vi "run_experiment_sCMOS_DAC_DEBUG_WORKING_INTER.vi"() -> ()   [LabVIEW 2015]
uses:
  <vilib>/DAQmx/read.llb/DAQmx Read (Analog 1D Wfm NChan NSamp).vi
  <vilib>/DAQmx/write.llb/DAQmx Write (Digital Bool 1Line 1Point).vi
  <vilib>/DAQmx/create/channels.llb/DAQmx Create Channel (DO-Digital Output).vi
  <vilib>/DAQmx/miscellaneous.llb/DAQmx Fill In Error Info.vi
  <vilib>/DAQmx/create/channels.llb/DAQmx Create Channel (AI-Voltage-Basic).vi
  <vilib>/DAQmx/configure/timing.llb/DAQmx Timing (Sample Clock).vi
panel:
  out "Display":T1(plugin-control)
  out "DAC Input":waveform(dbl)[](graph) caption="DAC Input Display"
  out "error out":errorcluster
  out "Current Stimulus Name":string
  out "Current Piezo Command":dynamicdata(graph)
  out "Acquiring Frames":bool
  out "Current Stim Duration":dbl
  out "Current Stimulus Save Path":path
  in  "Number Reps":dbl
  out "Experiment Path":path
  out "Timestamp":string
  out "Genotype":string
  out "Fly Name":string
  out "Experiment Name":string
  in  "Metadata Path":path
  out "Stimulus Files":path[](array[path])
  out "Num Stimuli":i32
  out "Protocol Name":string
  out "Protocol Rate":i32
  in  "Protocol Path":path
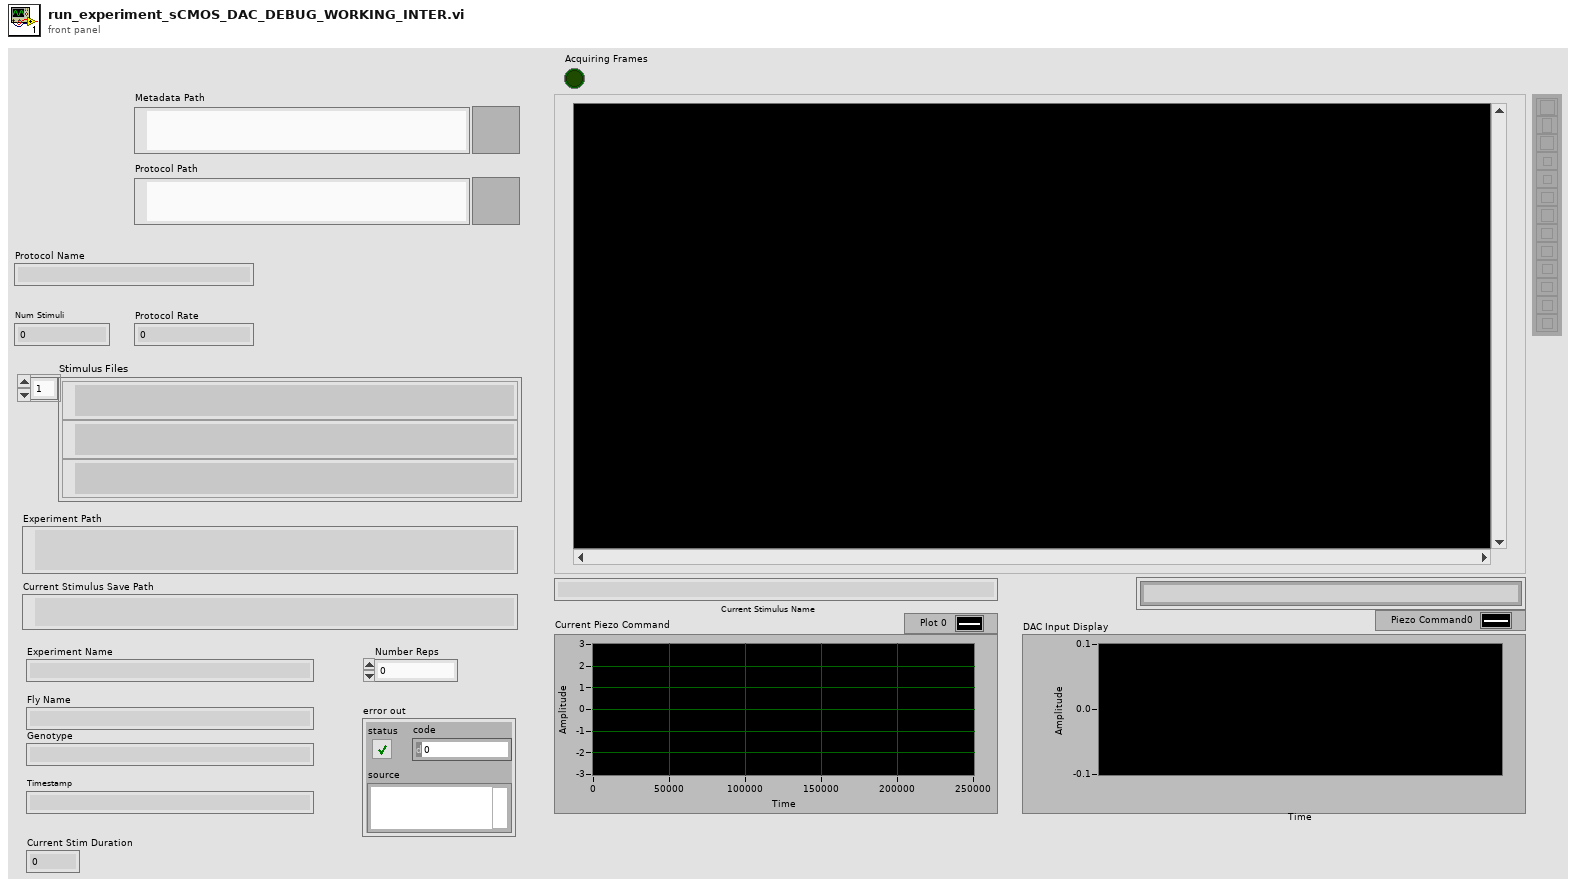
[diagram p1: front panel]
types:
  T1 = typedef "IMAQ Image.ctl" = refnum<image>
  T2 = cluster{"Value":i32, "Minimum":i32, "Maximum":i32, "Increment":i32}
  T3 = cluster{"height":u32, "width":u32, "datatype":u32}
  T4 = typedef "Image Type" = u32
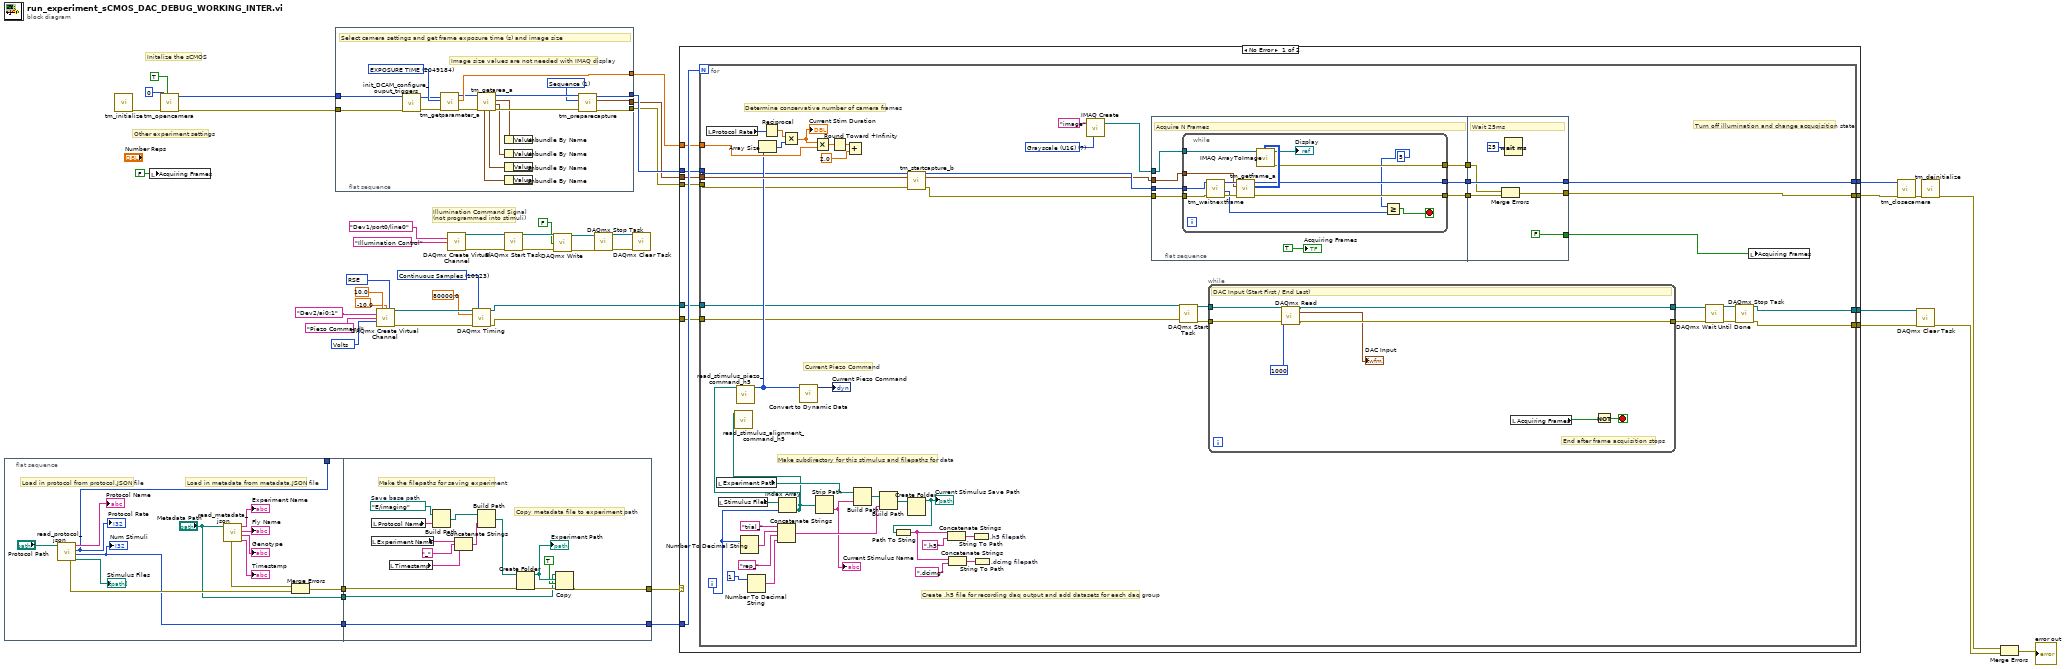
[diagram p0: block diagram]
diagram:
  w8 = 10083 items=["default"=-1, "RSE"=10083, "NRSE"=10078, "Differential"=10106, "Pseudodifferential"=12529] ("input terminal configuration")
  w9 = 10123 items=["Finite Samples"=10178, "Continuous Samples"=10123] ("sample mode")
  w10 = 10348 items=["Volts"=10348, "From Custom Scale"=10065] ("units")
  # "Other experiment settings"
  # "Initalize the sCMOS"
  # "Illumination Command Signal \n(not programmed into stimuli)"
  n1 = flat-sequence {
    tunnel: [w49] -> _
    tunnel: [w50] -> w21
    tunnel: ["Metadata Path"] -> w20
    tunnel: [w47] -> w19
    tunnel: [w74] -> w40
    tunnel: w21 -> [w62]
    tunnel: w20 -> [w61]
    tunnel: w19 -> [w74]
    tunnel: [w60] -> w18
    frame #0 {
      # "Load in metadata from metadata.JSON file"
      # "Load in protocol from protocol.JSON file"
      n2 = call "read_protocol_json.vi"("Path"="Protocol Path") -> ("stims"=→"Stimulus Files":path[], "n_stims"=w47:i32, "rate"=w49:i32, "protocol name"=→"Protocol Name":string, "error out"=w52:errorcluster)  [unwired: 6 in]
      "Protocol Rate" <- w49
      "Num Stimuli" <- w47
      n3 = call "read_metadata_json.vi"("Path"="Metadata Path") -> ("exp_time"=→"Timestamp":string, "genotype"=→"Genotype":string, "fly_name"=→"Fly Name":string, "exp_ name"=→"Experiment Name":string, "error out"=w51:errorcluster)  [unwired: 6 in]
      n4 = Merge Errors(w51, w52) -> (w50:errorcluster)
    }
    frame #1 {
      w69 = path "E:/imaging"  # Save base path
      # "Copy metadata file to experiment path"
      # "Make the filepaths for saving experiment"
      n5 = local read "Experiment Name"() -> (w66:string)
      n6 = local read "Protocol Name"() -> (w68:string)
      n7 = local read "Timestamp"() -> (w64:string)
      n8 = Build Path(base path=w69, name or relative path=w68) -> (appended path=w67:path)
      n9 = Concatenate Strings(w66, "_", w64) -> (w63:string)
      n10 = Build Path(base path=w67, name or relative path=w63) -> (appended path=w70:path)
      n11 = Create Folder(path (use dialog)=w70, error in=w62) -> (created path=w73:path, error out=w72:errorcluster)  [unwired: 1 in, 1 out]
      "Experiment Path" <- w73
      n12 = Copy(8:w72, 9:TRUE ("overwrite (F)"), 10:w73, 11:w61) -> (0:w60:errorcluster)  [unwired: 1 in, 2 out]
    }
  }
  n13 = call <userlib>:"tm_initialize.vi"() -> ("error out"=w43:errorcluster)  [unwired: 8 in, 3 out]
  n14 = local write "Acquiring Frames"(FALSE ("Acquiring Frames")) -> ()
  n15 = call <userlib>:"tm_opencamera.vi"("Force Open"=TRUE, "error in (no error)"=w43, "Camera Index"=0) -> ("error out"=w29:errorcluster, "Handle out"=w30:u32)  [unwired: 6 in, 1 out]
  n16 = flat-sequence {
    tunnel: [w88] -> w33
    tunnel: [w87] -> w24
    tunnel: [w86] -> w32
    tunnel: [w91] -> w31
    tunnel: w30 -> [w76]
    tunnel: w29 -> [w75]
    frame #0 {
      w77 = 1 items=["Snap", "Sequence"] ("Capture mode")
      w92 = u32 2049184 items=["SENSOR MODE"=4212128, "CCD MODE"=4212384, "READOUT MODE"=4211872, "ACTIVE VIEW INDEX"=4343136, "BITS PER CHANNEL"=4342976, "IMAGE PIXEL TYPE"=4343296, "BINNING"=4215968, "EXPOSURE TIME"=2049184, "CONTRAST GAIN"=3163312, "CONTRAST OFFSET"=3163328, "LIGHT MODE"=2114720, "SENSITIVITY"=2114992, "PHOTON IMAGING MODE"=2115200, "HIGH DYNAMIC RANGE MODE"=3163360, "WHITE BALANCE"=3163568, "TEMPERATURE"=2115232, "TEMPERATURE TARGET"=2115264, "SENSOR COOLER FAN"=2115296, "LINEBUNDLE HEIGHT"=4212192, "MECHANICAL SHUTTER"=2115488, "BACK FOCUS POSITION"=8422304, "TRIGGER CONNECTOR"=1066432, "TRIGGER SOURCE"=1066144, "OUTPUT TRIGGER SOURCE"=1852576, "TRIGGER GLOBAL EXPOSURE"=2049680, "FIRST TRIGGER BEHAVIOR"=2049696, "CHANNEL SYNC"=1852352, "READOUT DIRECTION"=4211904, "PRE HSYNC COUNT"=1852704] ("Parameter")
      # "Image size values are not needed with IMAQ display"
      # "Select camera settings and get frame exposure time (s) and image size"
      n17 = call "init_DCAM_configure_ouput_triggers.vi"("error in (no error)"=w75, "Handle in"=w76) -> ("error out"=w90:errorcluster, "Handle out"=w89:u32)  [unwired: 2 in]
      n18 = call <userlib>:"tm_getparameter_a.vi"("error in (no error)"=w90, "Parameter"=w92, "Handle in"=w89) -> ("error out"=w84:errorcluster, "Value out"=w91:dbl, "Handle out"=w85:u32)  [unwired: 6 in]
      n19 = call <userlib>:"tm_getarea_a.vi"("error in (no error)"=w84, "Handle in"=w85) -> ("error out"=w82:errorcluster, "V Offset"=w80:T2, "H Offset"=w81:T2, "Handle out"=w83:u32, "H Width"=w79:T2, "V Width"=w78:T2)  [unwired: 4 in]
      n20 = Unbundle By Name(w81) -> ()  [unwired: 1 out]
      n21 = Unbundle By Name(w80) -> ()  [unwired: 1 out]
      n22 = Unbundle By Name(w79) -> ()  [unwired: 1 out]
      n23 = Unbundle By Name(w78) -> ()  [unwired: 1 out]
      n24 = call <userlib>:"tm_preparecapture.vi"("error in (no error)"=w82, "Capture mode"=w77, "Handle in"=w83) -> ("error out"=w87:errorcluster, "Buffer Info"=w86:T3, "Handle out"=w88:u32)  [unwired: 5 in, 1 out]
    }
  }
  n25 = call-poly <vilib>:"DAQmx Create Virtual Channel.vi"("maximum value"=10.0, "minimum value"=-10.0, "input terminal configuration"=w8, "physical channels"=tag "Dev2/ai0:1" ("DAQmx Physical Channel"), "name to assign"="Piezo Command", "units"=w10) -> ("task out"=w16:refnum<k21>, "error out"=w17:errorcluster)  [unwired: 8 in]
  n26 = call-poly <vilib>:"DAQmx Create Virtual Channel.vi"("lines"=tag "Dev1/port0/line0" ("DAQmx Physical Channel"), "name to assign"="Illumination Control") -> ("task out"=w37:refnum<k21>, "error out"=w39:errorcluster)  [unwired: 12 in]
  n27 = call-poly <vilib>:"DAQmx Timing.vi"("task/channels in"=w16, "sample mode"=w9, "rate"=80000.0, "error in"=w17) -> ("task out"=w7:refnum<k21>, "error out"=w6:errorcluster)  [unwired: 10 in]
  n28 = call <vilib>:"DAQmx Start Task.vi"("task/channels in"=w37, "error in"=w39) -> ("task out"=w36:refnum<k21>, "error out"=w38:errorcluster)  [unwired: 12 in]
  n29 = call-poly <vilib>:"DAQmx Write.vi"("task/channels in"=w36, "data"=FALSE, "error in"=w38) -> ("task out"=w5:refnum<k21>, "error out"=w4:errorcluster)  [unwired: 10 in, 1 out]
  n30 = call <vilib>:"DAQmx Stop Task.vi"("task/channels in"=w5, "error in"=w4) -> ("task out"=w2:refnum<k21>, "error out"=w3:errorcluster)  [unwired: 12 in]
  n31 = call <vilib>:"DAQmx Clear Task.vi"("task in"=w2, "error in"=w3) -> ()  [unwired: 13 in, 1 out]
  n32 = case shown="No Error" w18 {
    tunnel: w40 -> [w103 _]
    tunnel: w31 -> [w102 _]
    tunnel: w33 -> [w101 w194]
    tunnel: w24 -> [w100 w193]
    tunnel: w32 -> [w99 _]
    tunnel: [w98 w193] -> w26
    tunnel: [w97 w194] -> w25
    tunnel: [w96 _] -> w23
    tunnel: [w95 _] -> w22
    tunnel: w7 -> [w94 _]
    tunnel: w6 -> [w93 _]
    frame No Error {
      n33 = for {
        N: w103 -> [_]
        tunnel: w102 -> [w140]
        tunnel: w101 -> [w104]
        tunnel: w100 -> [w105]
        tunnel: w99 -> [w128]
        tunnel: [w122] -> w98
        tunnel: [w121] -> w97
        tunnel: [w109] -> w96
        tunnel: [w108] -> w95
        tunnel: w94 -> [w107]
        tunnel: w93 -> [w106]
        i -> [w153]
        w117 = T4 7 items=["Grayscale (U8)", "Grayscale (I16)", "Grayscale (SGL)", "Complex (CSG)", "RGB (U32)", "HSL (U32)", "RGB (U64)", "Grayscale (U16)"] ("Image Type")
        # "Create .h5 file for recording daq output and add datasets for each daq group"
        # "Current Piezo Command"
        # "Turn off illumination and change acquqisition state"
        # "Determine conservative number of camera frames"
        # "Make subdirectory for this stimulus and filepaths for data"
        n34 = local read "Protocol Rate"() -> (w144:i32)
        n35 = local read "Experiment Path"() -> (w146:path)
        n36 = local read "Stimulus Files"() -> (w154:path[])
        n37 = Number To Decimal String(number=w153) -> (decimal integer string=w156:string)  [unwired: 1 in]
        n38 = Number To Decimal String(number=i16 1 ("width (-)")) -> (decimal integer string=w151:string)  [unwired: 1 in]
        n39 = Reciprocal(x=w144) -> (1/x=w142:dbl)
        n40 = Concatenate Strings("trial_", w156, "rep_", w151) -> (w147:string)
        n41 = Index Array(array=w154, index=w153) -> (element=w145:path)
        n42 = call "read_stimulus_alignment_command_h5.vi"("Path"=w145) -> ()  [unwired: 9 in, 2 out]
        n43 = call "read_stimulus_piezo_command_h5.vi"("Path"=w145) -> ("stimulus"=w114:i32[])  [unwired: 9 in, 1 out]
        n44 = Array Size(array=w114) -> (size(s)=w143:i32)
        n45 = Multiply(x=w142, y=w143) -> (x*y=w141:dbl)
        "Current Stim Duration" <- w141
        n46 = call "Convert to Dynamic Data"("Array"=w114) -> ("Dynamic Data Type"=→"Current Piezo Command":dynamicdata)  [unwired: 3 in]
        n47 = Multiply(x=w141, y=w140) -> (x*y=w139:dbl)
        n48 = Strip Path(path=w145) -> (name=w125:string)  [unwired: 1 out]
        "Current Stimulus Name" <- w125
        n49 = Round Toward +Infinity(x=w139) -> (ceil(x): smallest int >= x=w138:dbl)
        n50 = Add(x=w138, y=2.0) -> ()  [unwired: 1 out]
        n51 = Build Path(base path=w146, name or relative path=w125) -> (appended path=w148:path)
        n52 = Build Path(base path=w148, name or relative path=w147) -> (appended path=w149:path)
        n53 = call <userlib>:"tm_startcapture_b.vi"("error in (no error)"=w105, "Handle in"=w104) -> ("error out"=w130:errorcluster, "Handle out"=w129:u32)  [unwired: 8 in]
        n54 = Create Folder(path (use dialog)=w149) -> (created path=w136:path)  [unwired: 2 in, 2 out]
        "Current Stimulus Save Path" <- w136
        n55 = Path To String(path=w136) -> (string=w133:string)
        n56 = Concatenate Strings(w133, ".h5" ("string")) -> (w135:string)
        n57 = Concatenate Strings(w133, ".dcimg" ("string")) -> (w134:string)
        n58 = String To Path ".h5 filepath"(string=w135) -> ()  [unwired: 1 out]
        n59 = String To Path ".dcimg filepath"(string=w134) -> ()  [unwired: 1 out]
        n60 = call "IMAQ Create"("Image Name"="image", "Image Type"=w117) -> ("New Image"=w116:T1)  [unwired: 3 in, 1 out]
        n61 = flat-sequence {
          tunnel: [w160] -> w124
          tunnel: [w159] -> w123
          tunnel: [w157] -> w115
          tunnel: w130 -> [w163]
          tunnel: w128 -> [w162]
          tunnel: w129 -> [w161]
          tunnel: w116 -> [w158]
          tunnel: [FALSE] -> w127
          tunnel: w124 -> [w182]
          tunnel: w123 -> [w180]
          tunnel: [w181] -> w122
          tunnel: [w182] -> w121
          tunnel: w115 -> [w179]
          frame #0 {
            # "Acquire N Frames"
            n62 = while {
              tunnel: w163 -> [w176]
              tunnel: w162 -> [w175]
              tunnel: w161 -> [w174]
              tunnel: [w168] -> w160
              tunnel: [w167] -> w159
              tunnel: w158 -> [w172]
              tunnel: [w170] -> w157
              stop <- w173 stop-if-true
              n63 = call <userlib>:"tm_waitnextframe.vi"("error in (no error)"=w176, "Handle in"=w174) -> ("error out"=w178:errorcluster, "Frame Count"=w166:i32, "Handle out"=w177:u32)  [unwired: 6 in, 1 out]
              n64 = call <userlib>:"tm_getframe_a.vi"("error in (no error)"=w178, "Buffer Info"=w175, "Handle in"=w177) -> ("error out"=w167:errorcluster, "Data 16"=w171:u16[][], "Handle out"=w168:u32)  [unwired: 4 in, 2 out]
              n65 = call "IMAQ ArrayToImage"("Image Pixels (U16)"=w171, "Image"=w172) -> ("error out"=w170:errorcluster, "Image Out"=→"Display":T1)  [unwired: 8 in]
              n66 = Greater Or Equal?(x=5, y=w166) -> (x >= y?=w173:bool)
            }
            "Acquiring Frames" <- TRUE
          }
          frame #1 {
            # "Wait 25ms"
            n67 = Merge Errors(w179, w180) -> (w181:errorcluster)
            n68 = Wait (ms)(milliseconds to wait=u32 25) -> ()  [unwired: 1 out]
          }
        }
        n69 = call <vilib>:"DAQmx Start Task.vi"("task/channels in"=w107, "error in"=w106) -> ("task out"=w120:refnum<k21>, "error out"=w119:errorcluster)  [unwired: 12 in]
        n70 = while {
          tunnel: w119 -> [w188]
          tunnel: [w191] -> w110
          tunnel: w120 -> [w189]
          tunnel: [w190] -> w111
          stop <- w192 stop-if-true
          # "End after frame acquisition stops"
          # "DAC Input (Start First / End Last)"
          n71 = call-poly <vilib>:"DAQmx Read.vi"("task/channels in"=w189, "number of samples per channel"=1000, "error in"=w188) -> ("task out"=w190:refnum<k21>, "data"=→"DAC Input":waveform(dbl)[], "error out"=w191:errorcluster)  [unwired: 10 in]
          n72 = local read "Acquiring Frames"() -> (w186:bool)
          n73 = Not(x=w186) -> (.not. x?=w192:bool)
        }
        n74 = call <vilib>:"DAQmx Wait Until Done.vi"("task/channels in"=w111, "error in"=w110) -> ("task out"=w113:refnum<k21>, "error out"=w112:errorcluster)  [unwired: 12 in]
        n75 = call <vilib>:"DAQmx Stop Task.vi"("task/channels in"=w113, "error in"=w112) -> ("task out"=w108:refnum<k21>, "error out"=w109:errorcluster)  [unwired: 12 in]
        n76 = local write "Acquiring Frames"(w127) -> ()
      }
    }
    frame Error {
    }
  }
  n77 = call <userlib>:"tm_closecamera.vi"("error in (no error)"=w26, "Handle in"=w25) -> ("error out"=w28:errorcluster)  [unwired: 9 in]
  n78 = call <vilib>:"DAQmx Clear Task.vi"("task in"=w22, "error in"=w23) -> ("error out"=w1:errorcluster)  [unwired: 13 in]
  n79 = call <userlib>:"tm_deinitialize.vi"("error in (no error)"=w28) -> ("error out"=w27:errorcluster)  [unwired: 10 in]
  n80 = Merge Errors(w27, w1) -> (→"error out":errorcluster)
